vi "loadTest.vi"(8 "error in (no error)":errorcluster, 9 "Test":string, 10 "TestCase in":refnum<class "TestCase.lvclass">, 11 "TestLoader in":refnum<class "TestLoader.lvclass">) -> (0 "error out":errorcluster, 2 "TestSuite out":refnum<class "TestSuite.lvclass">, 3 "TestLoader out":refnum<class "TestLoader.lvclass">)   [LabVIEW 2011, in "TestLoader.lvclass"]
doc: "This VI runs a specified test method"
uses:
  TestLoader.lvclass
  TestSuite/TestSuite.lvclass
  TestCase/TestCase.lvclass
panel:
  # "JKI VI Tester for LabVIEW\nhttp://jkisoft.com/vi-tester\nCopyright (C) 2007-2009, JKI <info@jkisoft.com>\nALL RIGHTS RESERVED"
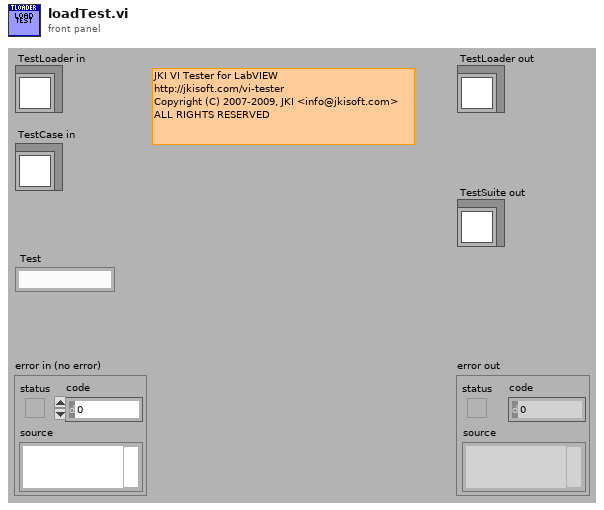
[diagram p1: front panel]
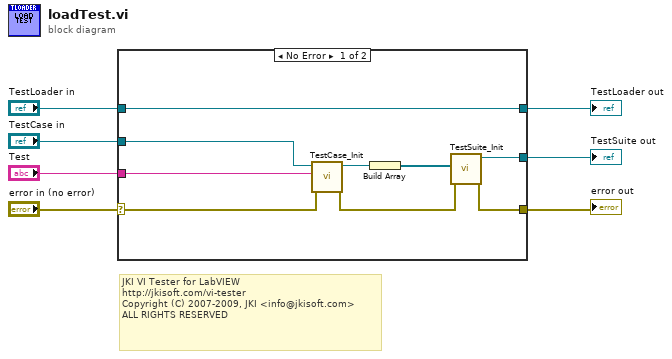
[diagram p0: block diagram]
diagram:
  # "JKI VI Tester for LabVIEW\nhttp://jkisoft.com/vi-tester\nCopyright (C) 2007-2009, JKI <info@jkisoft.com>\nALL RIGHTS RESERVED"
  n1 = case shown="No Error" "error in (no error)" {
    selector: "error in (no error)" -> [w9 w18]
    tunnel: [w13 w18] -> w6
    tunnel: [w16 w17] -> w4
    tunnel: "TestLoader in" -> [w16 w17]
    tunnel: "Test" -> [w12 _]
    tunnel: [w14 _] -> w2
    tunnel: "TestCase in" -> [w8 _]
    frame No Error {
      n2 = call "TestCase_Init.vi"("error in (no error)"=w9, "methodName (\"runTest\")"=w12, "TestCase in"=w8) -> ("error out"=w15:errorcluster, "TestCase out"=w11:refnum<class "TestCase.lvclass">)  [unwired: 7 in]
      n3 = Build Array(w11) -> (w10:refnum<class "TestCase.lvclass">[])
      n4 = call "TestSuite_Init.vi"("error in (no error)"=w15, "tests (none)"=w10) -> ("error out"=w13:errorcluster, "TestSuite out"=w14:refnum<class "TestSuite.lvclass">)  [unwired: 8 in]
    }
    frame Error {
    }
  }
  "error out" <- w6
  "TestLoader out" <- w4
  "TestSuite out" <- w2
